vi "Kafka_CloseConsumer.vi"(8 "error in (no error)":errorcluster, 11 "Consumer Handle":string="localhost:9092") -> (0 "error out":errorcluster, 3 "Consumer Handle":string)   [LabVIEW 2019, in "LVKafka.lvlib"]
uses:
  LVKafka.lvlib
  KafkaLVLib.dll
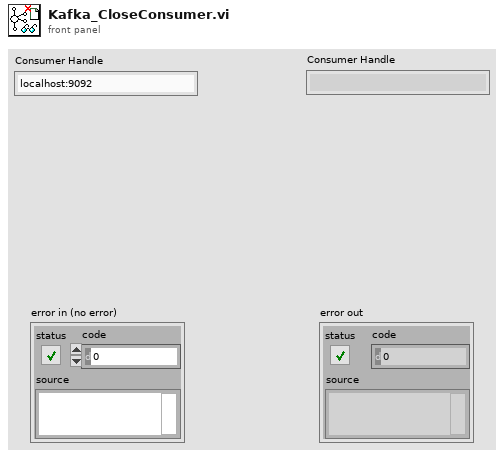
[diagram p1: front panel]
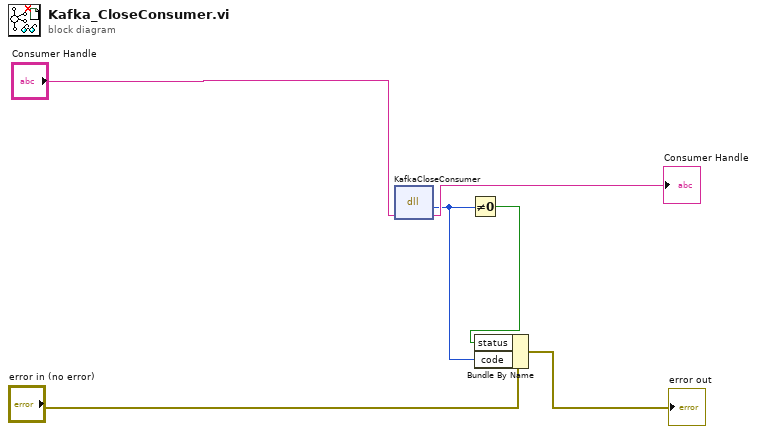
[diagram p0: block diagram]
diagram:
  n1 = dll-call lib="KafkaLVLib.*" fn="KafkaCloseConsumer"("consumerhandle"="Consumer Handle") -> ("error"=w1:i32, "consumerhandle"=→"Consumer Handle":string)  [unwired: 3 in, 2 out]
  n2 = Not Equal To 0?(x=w1) -> (x != 0?=w2:bool)
  n3 = Bundle By Name(cluster="error in (no error)", "status"=w2, "code"=w1) -> (→"error out":errorcluster)
